vi "savePharmaBotResults-v01loopReplicates.vi"(0 "controls array":refnum<vi>[](array[refnum]), 1 "protocol or memtest":enum16{"protocol", "memtest", "validation"}(ring), 2 "ExpPhase":string, 3 "which clamp":enum16{"VClamp", "IClamp"}(ring), 5 "protocol waveform":waveform(dbl), 7 "loop rec path in":path, 9 "protocol response":waveform(dbl), 11 "error in":errorcluster caption="error in (no error)", 12 "metadata to save":T1 {"cell stats"."STD" format="%010.2f"; "cell stats"."Variance" format="%010.2f"; "cell stats"."Rt (MOhms)" format="%010.2f"; "cell stats"."tau (ms)" format="%08.2g"; "cell stats"."Cm (pF)" format="%08.2f"; "cell stats"."Ra (MOhms)" format="%010.2f"; "cell stats"."Rm (MOhms)" format="%010.2f"; "cell stats"."Ihold (pA)" format="%010.2f"}, 13 "loop wave path in 2":path, 14 "Save to (folder dir)":path=path "C:/DATA/8-27-15 save func testing") -> (4 "controls array out":refnum<vi>[](array[refnum]), 6 "rec path out":path, 8 "wave path out 2":path, 15 "error out":errorcluster)   [LabVIEW 2019]
uses:
  autoWC/get_data_from_control_boolean.vi
  wc_protocol_v1.003 Folder/whole_cell_protocol/Controls/cell_stats-v02.ctl
  wc_protocol_v1.003 Folder/whole_cell_protocol/Controls/metadata_to_save.ctl
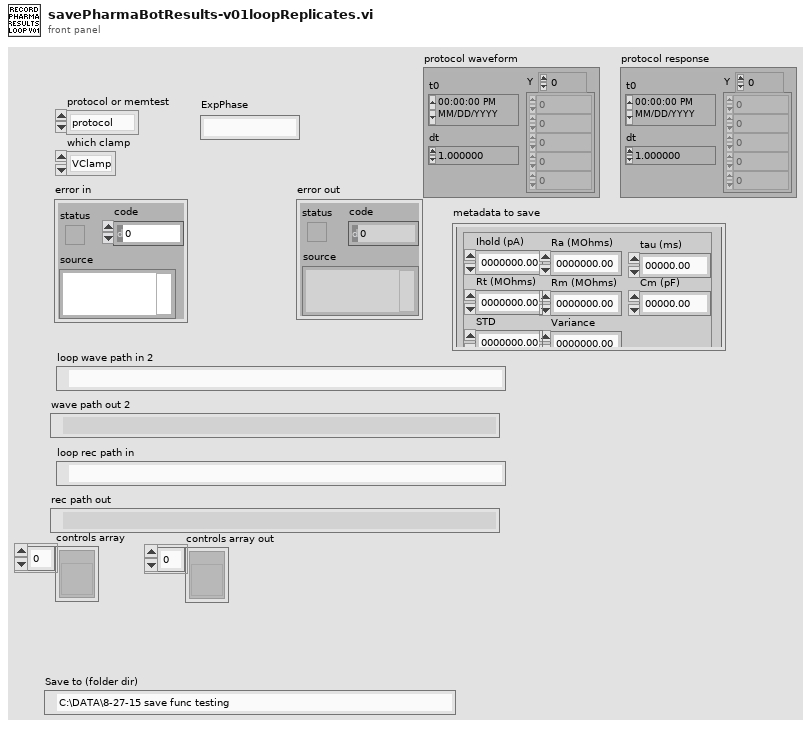
[diagram p1: front panel]
types:
  T1 = typedef "metadata_to_save.ctl" = cluster{"cell stats":T2}
  T2 = typedef "cell_stats-v02.ctl" = cluster{"Ihold (pA)":dbl, "Rm (MOhms)":dbl, "Ra (MOhms)":dbl, "Cm (pF)":dbl, "tau (ms)":dbl, "Rt (MOhms)":dbl, "Variance":dbl, "STD":dbl}
  T3 = enum16{"open", "replace", "create", "open or create", "replace or create", "replace or create with confirmation"}
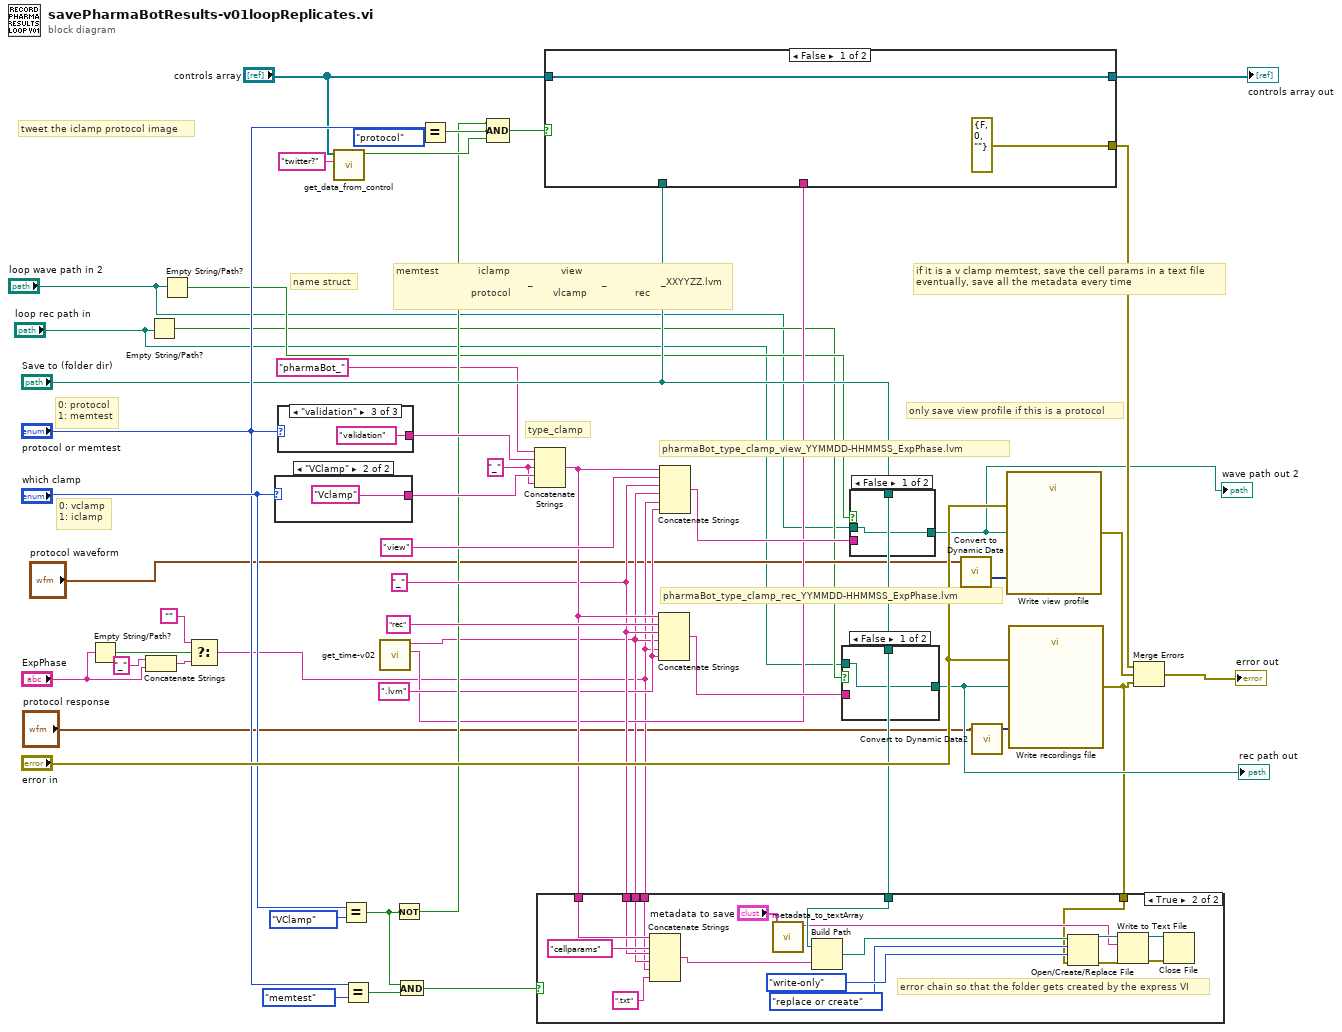
[diagram p0: block diagram]
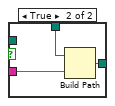
[diagram p2: hidden frame]
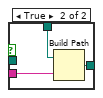
[diagram p3: hidden frame]
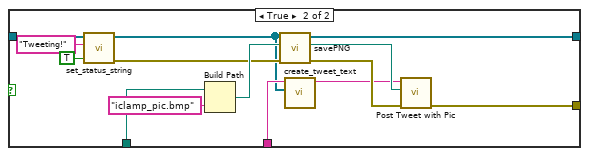
[diagram p4: hidden frame]
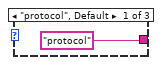
[diagram p6: hidden frame]
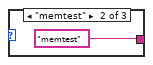
[diagram p7: hidden frame]
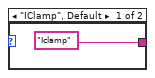
[diagram p8: hidden frame]
diagram:
  w17 = ".lvm" ("name or relative path")
  w32 = "_" ("string")
  w44 = "_" ("string")
  # "tweet the iclamp protocol image"
  # "if it is a v clamp memtest, save the cell params in a text file\neventually, save all the metadata every time"
  # "only save view profile if this is a protocol"
  # "pharmaBot_type_clamp_rec_YYMMDD-HHMMSS_ExpPhase.lvm"
  # "pharmaBot_type_clamp_view_YYMMDD-HHMMSS_ExpPhase.lvm"
  # "type_clamp"
  # "name struct"
  # "memtest             iclamp                 view            \n                                            _                       _                  _XXYYZZ.lvm\n                         protocol              vlcamp                rec"
  # "0: protocol\n1: memtest"
  # "0: vclamp\n1: iclamp"
  n1 = Empty String/Path?(string/path="ExpPhase") -> (empty?=w16:bool)
  n2 = Concatenate Strings("_" ("string"), "ExpPhase") -> (w13:string)
  n3 = Empty String/Path?(string/path="loop rec path in") -> (empty?=w3:bool)
  n4 = Empty String/Path?(string/path="loop wave path in 2") -> (empty?=w4:bool)
  n5 = Select(t="", s=w16, f=w13) -> (s? t:f=w8:string)
  n6 = case shown="\"VClamp\"" "which clamp" {
    tunnel: ["Iclamp" "Vclamp"] -> w45
    frame "IClamp", Default {
    }
    frame "VClamp" {
    }
  }
  n7 = case shown="\"validation\"" "protocol or memtest" {
    tunnel: ["protocol" "memtest" "validation"] -> w46
    frame "protocol", Default {
    }
    frame "memtest" {
    }
    frame "validation" {
    }
  }
  n8 = call-poly "get_data_from_control.vi"("control label"="twitter?", "controls array"="controls array") -> ("Boolean"=w23:bool)  [unwired: 8 in, 1 out]
  n9 = Equal?(x="which clamp", y=enum16{"VClamp", "IClamp"}."VClamp") -> (x = y?=w19:bool)
  n10 = Equal?(x="protocol or memtest", y=enum16{"protocol", "memtest"}."memtest") -> (x = y?=w21:bool)
  n11 = call "get_time-v02.vi"() -> ("time output"=w10:string, "pure text output"=w9:string)  [unwired: 10 in]
  n12 = Not(x=w19) -> (.not. x?=w18:bool)
  n13 = And(x=w19, y=w21) -> (x .and. y?=w34:bool)
  n14 = Equal?(x="protocol or memtest", y=enum16{"protocol", "memtest"}."protocol") -> (x = y?=w28:bool)
  n15 = Compound Arithmetic op=AND(w18, w28, w23) -> (w27:bool)
  n16 = Concatenate Strings("pharmaBot_" ("string"), w46, w44, w45, w44) -> (w33:string)
  n17 = case shown="False" w27 {
    tunnel: "controls array" -> [w57 w62]
    tunnel: [w57 w67] -> w26
    tunnel: "Save to (folder dir)" -> [_ w71]
    tunnel: [errorcluster {"status"=FALSE, "code"=0, "source"=""} ("error out") w65] -> w20
    tunnel: w10 -> [_ w64]
    frame False {
    }
    frame True {
      n18 = call "set_status_string.vi"("new line?"=TRUE, "status string in"="Tweeting!", "controls array"=w62) -> ("error out"=w61:errorcluster, "controls array out"=w58:refnum<vi>[])  [unwired: 7 in]
      n19 = Build Path(base path=w71, name or relative path="iclamp_pic.bmp") -> (appended path=w70:path)
      n20 = call "savePNG.vi"("error in"=w61, "image path in (.bmp)"=w70, "controls array in"=w58) -> ("error out"=w66:errorcluster, "image path out (.PNG)"=w68:path, "controls array out"=w67:refnum<vi>[])  [unwired: 6 in]
      n21 = call "create_tweet_text.vi"("controls array"=w58, "time string"=w64) -> ("tweet"=w63:string)  [unwired: 9 in]
      n22 = call "Post Tweet with Pic.vi"("error in"=w66, "Picture File (PNG, JPG, GIF)"=w68, "Tweet"=w63) -> ("error out"=w65:errorcluster)  [unwired: 8 in]
    }
  }
  "controls array out" <- w26
  n23 = Concatenate Strings(w33, "rec" ("name or relative path"), w32, w9, w8, w17) -> (w40:string)
  n24 = Concatenate Strings(w33, "view" ("name or relative path"), w32, w9, w8, w17) -> (w41:string)
  n25 = case shown="False" w3 {
    tunnel: w40 -> [_ w75]
    tunnel: [w72 w74] -> w39
    tunnel: "Save to (folder dir)" -> [_ w73]
    tunnel: "loop rec path in" -> [w72 _]
    frame False {
    }
    frame True {
      n26 = Build Path(base path=w73, name or relative path=w75) -> (appended path=w74:path)
    }
  }
  "rec path out" <- w39
  n27 = case shown="False" w4 {
    tunnel: w41 -> [_ w79]
    tunnel: "Save to (folder dir)" -> [_ w78]
    tunnel: [w76 w77] -> w5
    tunnel: "loop wave path in 2" -> [w76 _]
    frame False {
    }
    frame True {
      n28 = Build Path(base path=w78, name or relative path=w79) -> (appended path=w77:path)
    }
  }
  "wave path out 2" <- w5
  n29 = call "Convert to Dynamic Data"("Waveform"="protocol waveform") -> ("Dynamic Data Type"=w38:dynamicdata)  [unwired: 3 in]
  n30 = call "Convert to Dynamic Data2"("Waveform"="protocol response") -> ("Dynamic Data Type"=w50:dynamicdata)  [unwired: 3 in]
  n31 = call "Write view profile"("Signals"=w38, "error in (no error)"="error in", "Filename"=w5) -> ("error out"=w48:errorcluster)  [unwired: 14 in, 2 out]
  n32 = call "Write recordings file"("Signals"=w50, "error in (no error)"="error in", "Filename"=w39) -> ("error out"=w31:errorcluster)  [unwired: 14 in, 2 out]
  n33 = case shown="True" w34 {
    tunnel: "Save to (folder dir)" -> [_ w92]
    tunnel: w33 -> [_ w90]
    tunnel: w32 -> [_ w88]
    tunnel: w9 -> [_ w87]
    tunnel: w31 -> [_ w82]
    tunnel: w8 -> [_ w81]
    frame False {
    }
    frame True {
      # "error chain so that the folder gets created by the express VI"
      n34 = Concatenate Strings(w90, "cellparams" ("name or relative path"), w88, w87, w81, ".txt" ("name or relative path")) -> (w91:string)
      n35 = call "metadata_to_textArray.vi"("metadata to save"="metadata to save") -> ("xml string out"=w85:string)  [unwired: 10 in]
      n36 = Build Path(base path=w92, name or relative path=w91) -> (appended path=w93:path)
      n37 = Open/Create/Replace File(file path (use dialog)=w93, error in=w82, operation (0:open)=T3."replace or create", access (0:read/write)=enum16{"read/write", "read-only", "write-only"}."write-only") -> (refnum out=w94:refnum<file>, error out=w96:errorcluster)  [unwired: 2 in, 1 out]
      n38 = Write to Text File(file (use dialog)=w94, text=w85, error in=w96) -> (refnum out=w84:refnum<file>, error out=w95:errorcluster)  [unwired: 1 in, 1 out]
      n39 = Close File(refnum=w84, error in=w95) -> ()  [unwired: 2 out]
    }
  }
  n40 = Merge Errors(w20, w48, w31) -> (→"error out":errorcluster)
